vi "Scan for Pumps.vi"(8 "error in (no error)":errorcluster, 11 "ASIA Pump #":i32) -> (0 "error out":errorcluster, 2 "pumpCnt":u32, 3 "ASIA Pump #":i32)   [LabVIEW 2018, in "ASIA Pump.lvlib" / "ASIA Support VIs.lvlib"]
uses:
  ASIA Support VIs.lvlib
  Third Party Drivers/4600031 - Version 1.2-Asia Pump Drivers/AsiaPumpInterface.dll
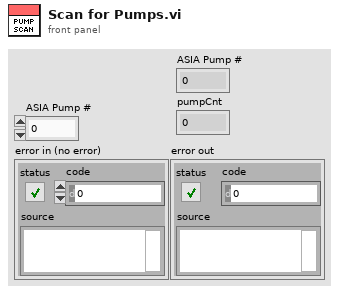
[diagram p1: front panel]
types:
  T1 = cluster{"Busy":bool, "PumpCnt":dbl, "RemoteEntered":bool, "OverpressureSet":bool}[]
  T2 = cluster{"Busy":bool, "PumpCnt":dbl, "RemoteEntered":bool, "OverpressureSet":bool}
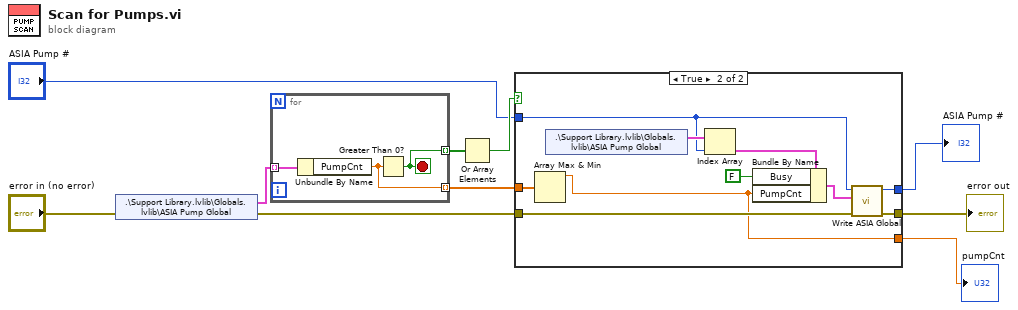
[diagram p0: block diagram]
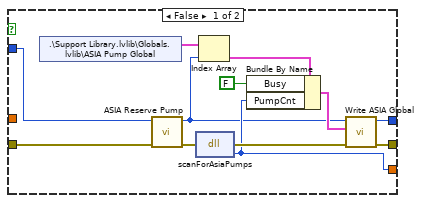
[diagram p2: hidden frame]
diagram:
  n1 = shared-variable ".\\Support Library.lvlib\\Globals.lvlib\\ASIA Pump Global"(error in="error in (no error)") -> (w10:T1, error out=w1:errorcluster)
  n2 = for {
    tunnel: w10 -> [w13] mode=indexing
    tunnel: [w12] -> w9 mode=indexing
    tunnel: [w11] -> w4 mode=indexing
    stop <- w12 stop-if-true
    n3 = Unbundle By Name(w13) -> ("PumpCnt"=w11:dbl)
    n4 = Greater Than 0?(x=w11) -> (x > 0?=w12:bool)
  }
  n5 = Or Array Elements(Boolean array=w9) -> (logical OR=w8:bool)
  n6 = case shown="True" w8 {
    tunnel: w1 -> [w23 w32]
    tunnel: "ASIA Pump #" -> [w22 w27]
    tunnel: [w21 w31] -> w3
    tunnel: [w20 w30] -> w6
    tunnel: [w17 w26] -> w5
    tunnel: w4 -> [_ w34]
    frame False {
      n7 = shared-variable ".\\Support Library.lvlib\\Globals.lvlib\\ASIA Pump Global"() -> (w16:T1)  [unwired: 1 in, 1 out]
      n8 = call "ASIA Reserve Pump.vi"("error in (no error)"=w23, "ASIA Pump #"=w22) -> ("error out"=w25:errorcluster, "ASIA Pump #"=w15:i32)  [unwired: 8 in]
      n9 = dll-call lib="C:/Users/FAST Lab/Documents/LabVIEW Data/Projects/Pfizer Timed Seq/Third Party Drivers/4600031 - Version 1.2-Asia Pump Drivers/AsiaPumpInterface.dll" fn="scanForAsiaPumps"(error in=w25) -> (error out=w24:errorcluster, "pumpCnt"=w17:u32)  [unwired: 2 in, 1 out]
      n10 = Index Array(array=w16, index=w15) -> (element=w14:T2)
      n11 = Bundle By Name(cluster=w14, "Busy"=FALSE, "PumpCnt"=w17) -> (w18:T2)
      n12 = call "Write ASIA Global.vi"("error in (no error)"=w24, "ASIA Global"=w18, "Pump Number"=w15) -> ("error out"=w21:errorcluster, "Pump Number"=w20:i32)  [unwired: 7 in]
    }
    frame True {
      n13 = Array Max & Min(array=w34) -> (max value=w26:dbl)  [unwired: 3 out]
      n14 = shared-variable ".\\Support Library.lvlib\\Globals.lvlib\\ASIA Pump Global"() -> (w29:T1)  [unwired: 1 in, 1 out]
      n15 = Index Array(array=w29, index=w27) -> (element=w28:T2)
      n16 = Bundle By Name(cluster=w28, "Busy"=FALSE, "PumpCnt"=w26) -> (w33:T2)
      n17 = call "Write ASIA Global.vi"("error in (no error)"=w32, "ASIA Global"=w33, "Pump Number"=w27) -> ("error out"=w31:errorcluster, "Pump Number"=w30:i32)  [unwired: 7 in]
    }
  }
  "ASIA Pump #" <- w6
  "pumpCnt" <- w5
  "error out" <- w3
